vi "VFD Close.vi"(8 "error In":errorcluster) -> (0 "error out":errorcluster)   [LabVIEW 2026, in "VFD Library.lvlib"]
uses:
  VFD Library.lvlib
  Private/State Selection FGV.ctl
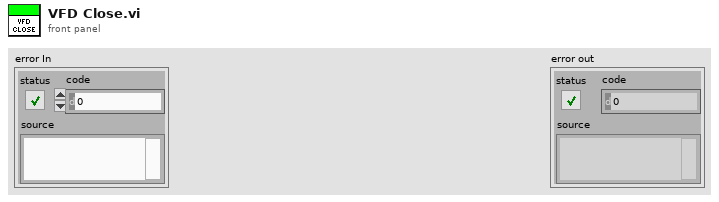
[diagram p1: front panel]
types:
  T1 = typedef "State Selection FGV.ctl" = enum16{"Initilize", "Write Reg", "Write Multiple Reg", "Read Reg", "Write Coil", "Read Coil", "Reset", "Close"}
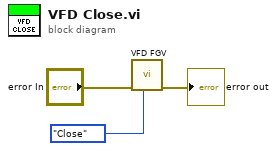
[diagram p0: block diagram]
diagram:
  n1 = call "VFD FGV.vi"("State"=State_Selection_FGV."Close", "error In"="error In") -> ("error out"=→"error out":errorcluster)  [unwired: 7 in, 2 out]
